vi "ep_Parse Section Headers.vi"(10 "raw section headers":string[](array[string]), 11 "manufacturer name":string) -> (2 "manufacturer/section names":string[][](array[string]), 3 "manufacturer names":string[](array[string]))   [LabVIEW 2011, in "NI_EP_COMTRADE.lvlib"]
uses:
  <vilib>/addons/Electrical Power/File IO/NI_EP_COMTRADE.lvlib
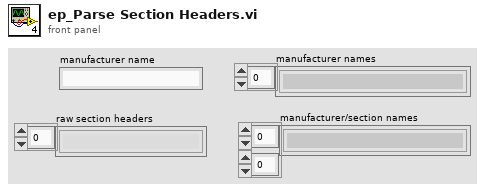
[diagram p1: front panel]
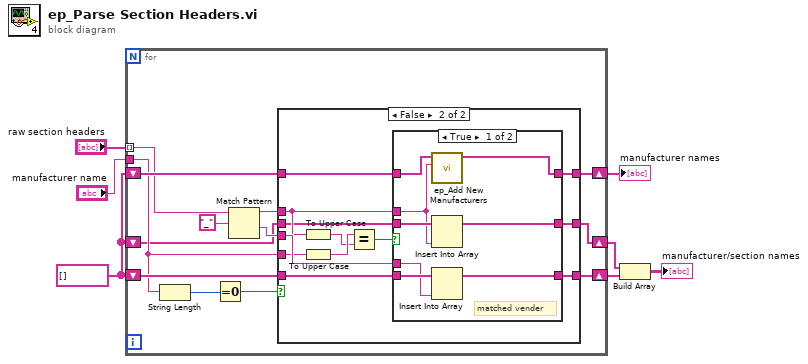
[diagram p0: block diagram]
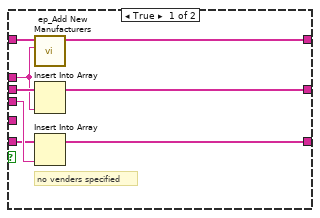
[diagram p2: hidden frame]
diagram:
  w1 = string[] [] ("Array 3")
  n1 = for {
    tunnel: "raw section headers" -> [w17] mode=indexing
    shift-right: [w13] -> w3
    shift-left: w1 -> [w18]
    tunnel: "manufacturer name" -> [w10]
    shift-right: [w12] -> w5
    shift-left: w1 -> [w11]
    shift-right: [w8] -> w2
    shift-left: w1 -> [w9]
    n2 = String Length(string=w10) -> (length=w20:i32)
    n3 = Equal To 0?(x=w20) -> (x = 0?=w19:bool)
    n4 = Match Pattern(string=w17, regular expression="_" ("search string/char (-)")) -> (before substring=w15:string, after substring=w14:string)  [unwired: 1 in, 2 out]
    n5 = case shown="False" w19 {
      tunnel: w18 -> [w25 w38]
      tunnel: w15 -> [w22 w33]
      tunnel: w14 -> [w28 w35]
      tunnel: [w24 w39] -> w13
      tunnel: [w26 w37] -> w12
      tunnel: w11 -> [w27 w36]
      tunnel: w10 -> [_ w34]
      tunnel: w9 -> [w23 w30]
      tunnel: [w21 w29] -> w8
      frame True {
        # "no venders specified"
        n6 = call <vilib>:"ep_Add New Manufacturers.vi"("manufacturer"=w22, "manufacturers input"=w25) -> ("manufacturer output"=w24:string[])  [unwired: 9 in]
        n7 = Insert Into Array(array=w23, new element=w22) -> (w21:string[])  [unwired: 1 in]
        n8 = Insert Into Array(array=w27, new element=w28) -> (w26:string[])  [unwired: 1 in]
      }
      frame False {
        n9 = To Upper Case(1:w33) -> (0:w31:string)
        n10 = To Upper Case(1:w34) -> (0:w32:string)
        n11 = Equal?(x=w32, y=w31) -> (x = y?=w40:bool)
        n12 = case shown="True" w40 {
          tunnel: [w45 w50] -> w39
          tunnel: w38 -> [w44 w50]
          tunnel: [w48 w51] -> w37
          tunnel: w36 -> [w47 w51]
          tunnel: w35 -> [w46 _]
          tunnel: w33 -> [w42 _]
          tunnel: w30 -> [w43 w49]
          tunnel: [w41 w49] -> w29
          frame True {
            # "matched vender"
            n13 = call <vilib>:"ep_Add New Manufacturers.vi"("manufacturer"=w42, "manufacturers input"=w44) -> ("manufacturer output"=w45:string[])  [unwired: 9 in]
            n14 = Insert Into Array(array=w43, new element=w42) -> (w41:string[])  [unwired: 1 in]
            n15 = Insert Into Array(array=w47, new element=w46) -> (w48:string[])  [unwired: 1 in]
          }
          frame False {
            # "no matched vender"
          }
        }
      }
    }
  }
  "manufacturer names" <- w3
  n16 = Build Array(w2, w5) -> (→"manufacturer/section names":string[][])
